vi "n set wobbel xy.vi"(7 "frequency":dbl, 8 "error in (no error)":errorcluster, 9 "trans_wob":u16, 10 "long_wob":u16, 11 "n":u16) -> (0 "error out":errorcluster)   [LabVIEW 2015, in "SCANalone4x64.lvlib"]
doc: "__declspec(dllimport) void __stdcall n_set_wobbel_xy(unsigned short n, unsigned short long_wob, unsigned short trans_wob, double frequency);"
uses:
  <userlib>/SCANalone4x64/SCANalone4x64.lvlib
  <userlib>/SCANalone4x64/SCANalone4x64.dll
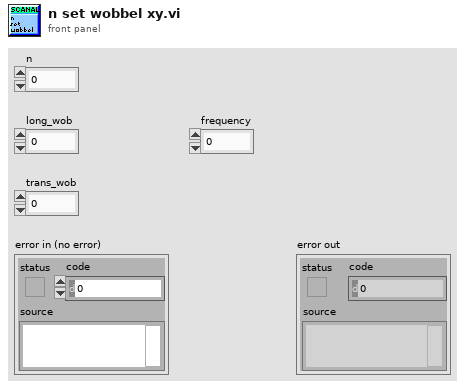
[diagram p1: front panel]
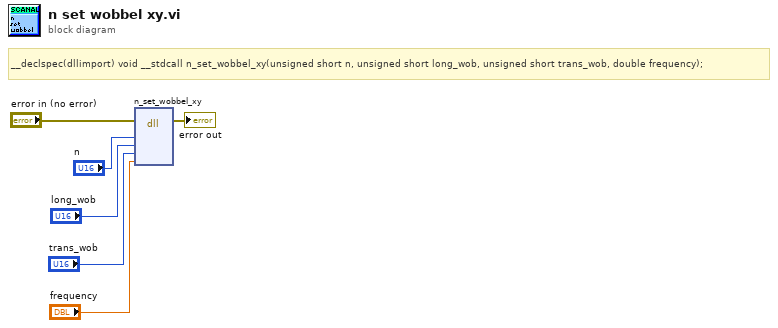
[diagram p0: block diagram]
diagram:
  # "__declspec(dllimport) void __stdcall n_set_wobbel_xy(unsigned short n, unsigned short long_wob, unsigned short trans_wob, double frequency);"
  n1 = dll-call lib="C:/Program Files/National Instruments/LabVIEW 2015/user.lib/SCANalone4x64/SCANalone4x64.*" fn="n_set_wobbel_xy"(error in="error in (no error)", "n"="n", "long_wob"="long_wob", "trans_wob"="trans_wob", "frequency"="frequency") -> (error out=→"error out":errorcluster)  [unwired: 7 in, 1 out]
